vi "Update Selected Waveform UI.vi"(8 "error in":errorcluster, 10 "Waveforms UI Ctrl Ref":T2, 11 "Waveform Meas Config Ctrl Ref":T1) -> (0 "error out":errorcluster)   [LabVIEW 2025, in "Fgen Script Mode UI.lvlib"]
uses:
  Fgen Script Mode UI.lvlib
  Typedef/Waveforms UI Ctrl Ref.ctl
  Typedef/Waveform Meas Config Ctrl Ref.ctl
  Typedef/Wfm Typedef.ctl
  <vilib>/ErrorRing/Error Ring.xnode
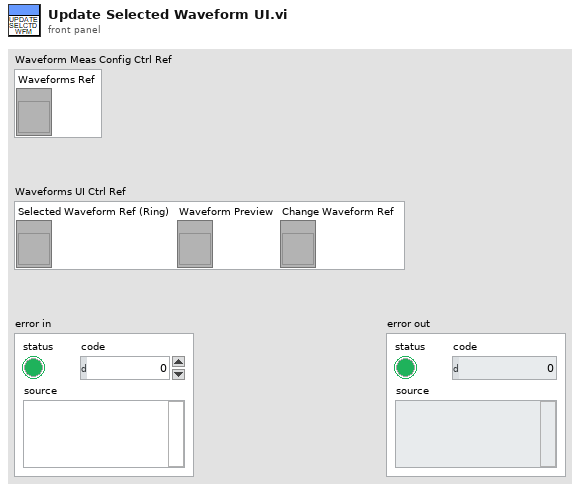
[diagram p1: front panel]
types:
  T1 = typedef "Fgen Script Mode UI.lvlib/Waveform Meas Config Ctrl Ref.ctl" = cluster{"Waveforms Ref":refnum<vi>}
  T2 = typedef "Fgen Script Mode UI.lvlib/Waveforms UI Ctrl Ref.ctl" = cluster{"Selected Waveform Ref (Ring)":refnum<vi>, "Waveform Preview":refnum<vi>, "Change Waveform Ref":refnum<vi>}
  T3 = enum8{"Enabled", "Disabled", "Disabled and Grayed Out"}
  T4 = typedef "Fgen Script Mode UI.lvlib/Wfm Typedef.ctl" = cluster{"Name":string, "Path":string, "Grp":string, "Chn":string}
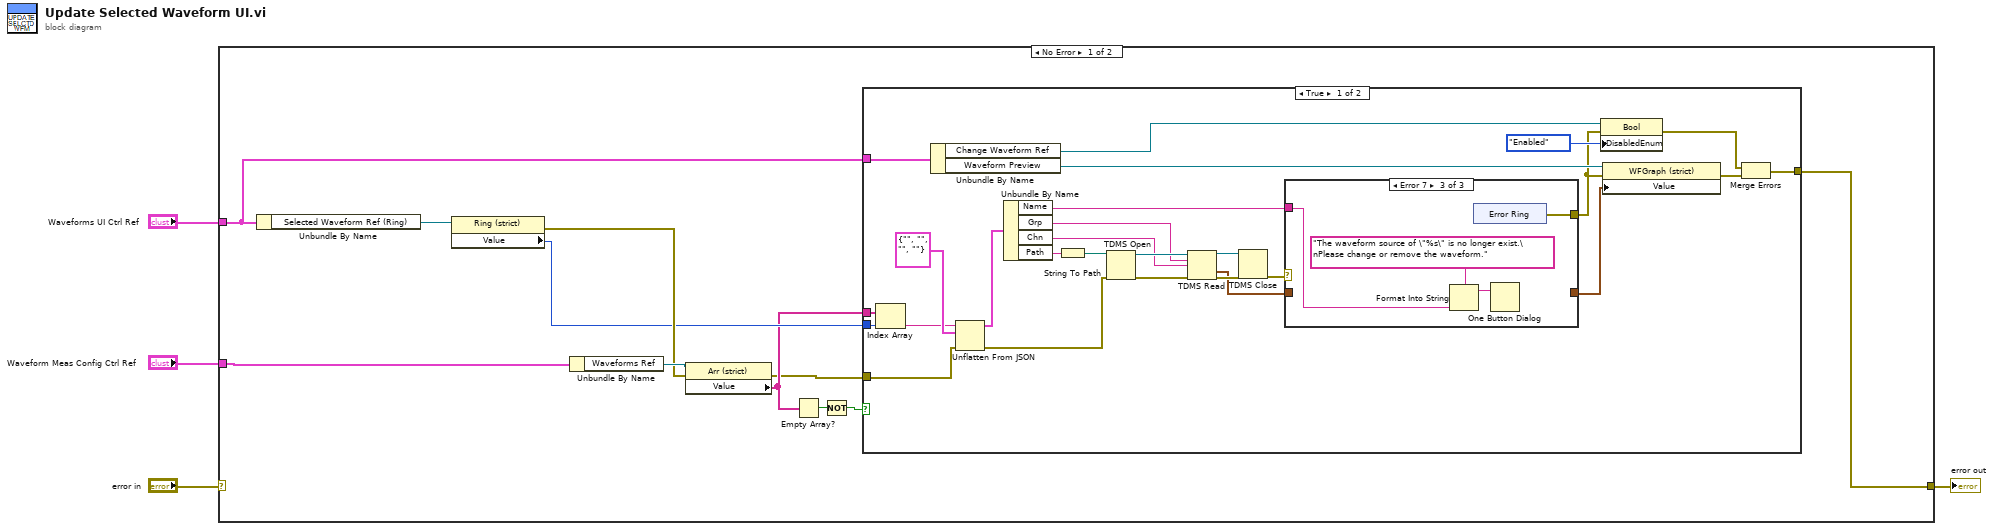
[diagram p0: block diagram]
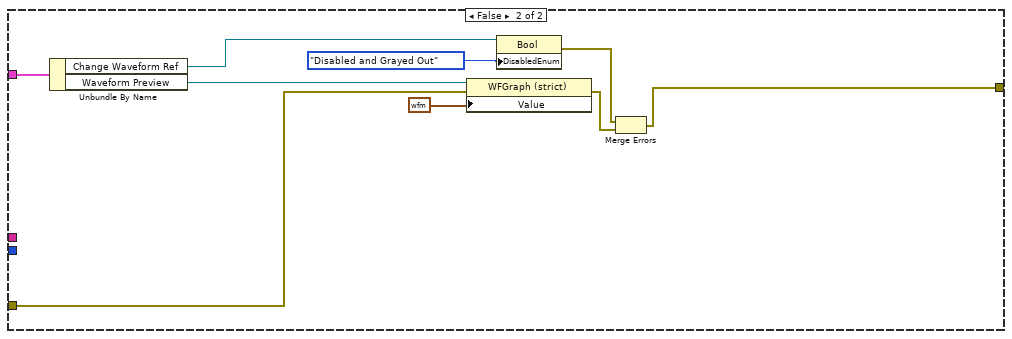
[diagram p4: hidden frame]
diagram:
  n1 = case shown="No Error" "error in" {
    selector: "error in" -> [_ w60]
    tunnel: [w5 w60] -> w3
    tunnel: "Waveform Meas Config Ctrl Ref" -> [w12 _]
    tunnel: "Waveforms UI Ctrl Ref" -> [w6 _]
    frame No Error {
      n2 = Unbundle By Name(w6) -> ("Selected Waveform Ref (Ring)"=w15:refnum<vi>)
      n3 = property class="Ring (strict)"(reference=w15) -> (error out=w13:errorcluster, "Value"=w11:u16)  [unwired: 1 in, 1 out]
      n4 = Unbundle By Name(w12) -> ("Waveforms Ref"=w14:refnum<vi>)
      n5 = property class="Arr (strict)"(reference=w14, error in=w13) -> (error out=w8:errorcluster, "Value"=w10:string[])  [unwired: 1 out]
      n6 = Empty Array?(array=w10) -> (empty?=w9:bool)
      n7 = Not(x=w9) -> (.not. x?=w7:bool)
      n8 = case shown="True" w7 {
        tunnel: w11 -> [w42 _]
        tunnel: w10 -> [w41 _]
        tunnel: w8 -> [w38 w59]
        tunnel: [w22 w53] -> w5
        tunnel: w6 -> [w27 w58]
        frame True {
          n9 = Index Array(array=w41, index=w42) -> (element=w39:string)
          n10 = Unbundle By Name(w27) -> ("Change Waveform Ref"=w23:refnum<vi>, "Waveform Preview"=w26:refnum<vi>)
          n11 = Unflatten From JSON(JSON string=w39, type and defaults=T4 {"Name"="", "Path"="", "Grp"="", "Chn"=""} ("Waveform"), error in (no error)=w38) -> (value=w37:T4, error out=w32:errorcluster)  [unwired: 4 in]
          n12 = Unbundle By Name(w37) -> ("Name"=w16:string, "Grp"=w31:string, "Chn"=w30:string, "Path"=w36:string)
          n13 = String To Path(string=w36) -> (path=w35:path)
          n14 = TDMS Open(8:w32, 11:w35) -> (0:w33:errorcluster, 3:w34:refnum<k34>)  [unwired: 5 in]
          n15 = TDMS Read(0:w34, 5:w31, 7:w30, 11:w33) -> (4:w28:refnum<k34>, 10:w19:waveform(dbl), 15:w29:errorcluster)  [unwired: 4 in, 3 out]
          n16 = TDMS Close(8:w29, 11:w28) -> (0:w20:errorcluster)  [unwired: 1 out]
          n17 = case shown="Error 7" w20 {
            selector: w20 -> [w44 w45 _]
            tunnel: [w44 w45 w49] -> w17
            tunnel: w19 -> [w43 _ _]
            tunnel: [w43 _ _] -> w18
            tunnel: w16 -> [_ _ w46]
            frame No Error {
            }
            frame Default {
            }
            frame Error {
              n18 = Format Into String(format string="The waveform source of \"%s\" is no longer exist.\nPlease change or remove the waveform.", w46) -> (resulting string=w48:string)  [unwired: 2 in, 1 out]
              n19 = xnode "Error Ring"() -> ("error out"=w49:errorcluster)
              n20 = One Button Dialog(message=w48) -> ()  [unwired: 1 in, 1 out]
            }
          }
          n21 = property class="Bool"(reference=w23, error in=w17, "DisabledEnum"=T3."Enabled" ("Disabled")) -> (error out=w21:errorcluster)  [unwired: 1 out]
          n22 = property class="WFGraph (strict)"(reference=w26, error in=w17, "Value"=w18) -> (error out=w25:errorcluster)  [unwired: 1 out]
          n23 = Merge Errors(w21, w25) -> (w22:errorcluster)
        }
        frame False {
          n24 = Unbundle By Name(w58) -> ("Change Waveform Ref"=w52:refnum<vi>, "Waveform Preview"=w57:refnum<vi>)
          n25 = property class="WFGraph (strict)"(reference=w57, error in=w59, "Value"=waveform(dbl) {"t0"=timestamp(0 s since 1904-01-01), "dt"=1.0, "Y"=[]}) -> (error out=w56:errorcluster)  [unwired: 1 out]
          n26 = property class="Bool"(reference=w52, "DisabledEnum"=T3."Disabled and Grayed Out" ("Disabled")) -> (error out=w51:errorcluster)  [unwired: 1 in, 1 out]
          n27 = Merge Errors(w51, w56) -> (w53:errorcluster)
        }
      }
    }
    frame Error {
    }
  }
  "error out" <- w3
